vi "_TangoAttributeConfigEventHandler.vi"(3 "error in":errorcluster, 4 "timeout (ms)":i32=1000, 5 "attribute config event ref":T6) -> (0 "error out":errorcluster, 1 "attribute info":T1, 2 "event timeout":bool)   [LabVIEW 2014, in "tango.lvlib"]
uses:
  tango.lvlib
  Common VIs/Typedefs/_AttributeConfigEventRef.ctl
  Common VIs/Typedefs/_AttributeInfo_t.ctl
  Common VIs/Typedefs/_AttributeAccess_t.ctl
  Common VIs/Typedefs/_AttributeFormat_t.ctl
  Common VIs/Typedefs/_TangoDataType_t.ctl
  Common VIs/Typedefs/_AttributeLevel_t.ctl
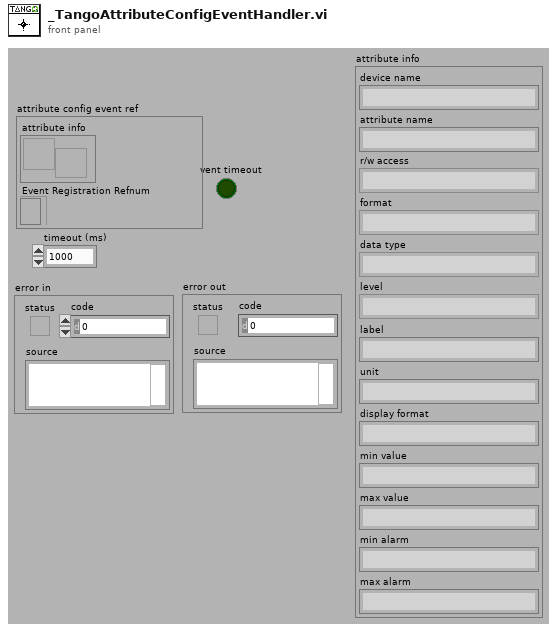
[diagram p1: front panel]
types:
  T1 = typedef "tango.lvlib/_AttributeInfo_t.ctl" = cluster{"device name":string, "attribute name":string, "r/w access":T2, "format":T3, "data type":T4, "level":T5, "label":string, "unit":string, "display format":string, "min value":string, "max value":string, "min alarm":string, "max alarm":string}
  T2 = typedef "tango.lvlib/_AttributeAccess_t.ctl" = enum16{"READ", "READ_WITH_WRITE", "WRITE", "READ_WRITE", "UNKNOWN_ACCESS_TYPE"}
  T3 = typedef "tango.lvlib/_AttributeFormat_t.ctl" = enum16{"SCALAR", "SPECTRUM", "IMAGE", "UNKNOWN_FORMAT"}
  T4 = typedef "tango.lvlib/_TangoDataType_t.ctl" = enum16{"VOID", "BOOLEAN", "SHORT", "LONG", "FLOAT", "DOUBLE", "USHORT", "ULONG", "STRING", "CHAR_ARRAY", "SHORT_ARRAY", "LONG_ARRAY", "FLOAT_ARRAY", "DOUBLE_ARRAY", "USHORT_ARRAY", "ULONG_ARRAY", "STRING_ARRAY", "LONG_STRING_ARRAY", "DOUBLE_STRING_ARRAY", "STATE", "CONST_STRING", "BOOLEAN_ARRAY", "UCHAR", "LONG64", "ULONG64", "LONG64_ARRAY", "ULONG64_ARRAY", "INT (not supported)", "ENCODED (not supported)", "ENUM", "PIPE_BLOB (not supported)", "STATE_ARRAY", "UNKNOW_DATA_TYPE"}
  T5 = typedef "tango.lvlib/_AttributeLevel_t.ctl" = enum16{"OPERATOR", "EXPERT", "UNKNOWN_LEVEL"}
  T6 = typedef "tango.lvlib/_AttributeConfigEventRef.ctl" = cluster{"attribute info":refnum<user-event>, "Event Registration Refnum":refnum<event-registration>}
  T7 = cluster{"device name":string, "attribute name":string, "r/w access":T2, "format":T3, "data type":T4, "level":T5, "label":string, "unit":string, "display format":string, "min value":string, "max value":string, "min alarm":string, "max alarm":string}
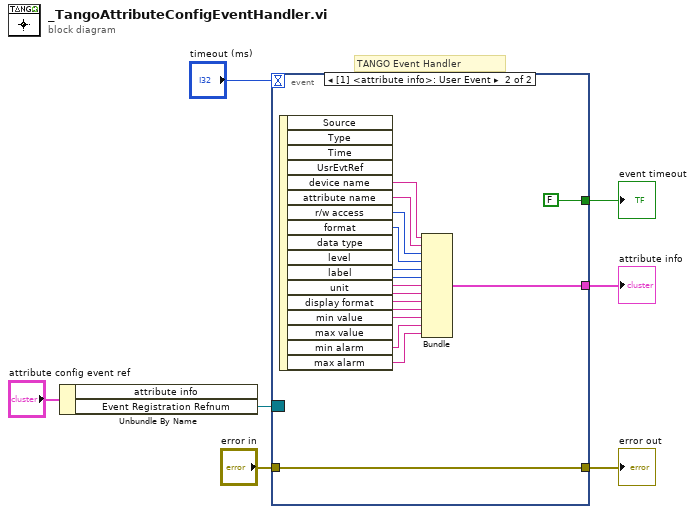
[diagram p0: block diagram]
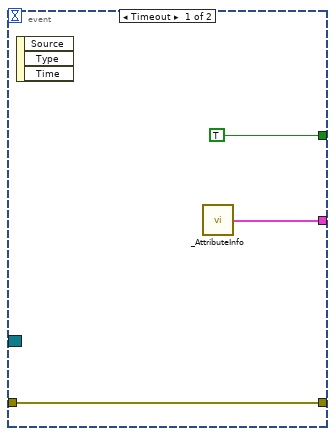
[diagram p2: hidden frame]
diagram:
  # "TANGO Event Handler"
  n1 = Unbundle By Name("attribute config event ref") -> ("Event Registration Refnum"=w3:refnum<event-registration>)  [unwired: 1 out]
  n2 = event shown="[1] <attribute info>: User Event" {
    selector: w3 -> [_ _]
    dyn-events: _ -> [_ _]
    timeout: "timeout (ms)" -> [_ _]
    tunnel: [TRUE FALSE] -> w7
    tunnel: "error in" -> [w9 w13]
    tunnel: [w9 w13] -> w5
    tunnel: [w8 w12] -> w2
    event Timeout {
      n3 = event-data() -> ()  [unwired: 1 in, 3 out]
      n4 = call "_AttributeInfo.vi"() -> ("attribute info"=w8:T1)  [unwired: 15 in]
    }
    event User Event {
      n5 = event-data() -> ("device name"=w26:string, "attribute name"=w25:string, "r/w access"=w24:T2, "format"=w23:T3, "data type"=w22:T4, "level"=w21:T5, "label"=w20:string, "unit"=w19:string, "display format"=w18:string, "min value"=w17:string, "max value"=w16:string, "min alarm"=w15:string, "max alarm"=w14:string)  [unwired: 1 in, 4 out]
      n6 = Bundle("device name"=w26, "attribute name"=w25, "r/w access"=w24, "format"=w23, "data type"=w22, "level"=w21, "label"=w20, "unit"=w19, "display format"=w18, "min value"=w17, "max value"=w16, "min alarm"=w15, "max alarm"=w14) -> (w12:T7)  [unwired: 1 in]
    }
  }
  "event timeout" <- w7
  "error out" <- w5
  "attribute info" <- w2
